vi "Cfg from FP.vi"(8 "error in (no error)":errorcluster, 11 "Measure Object in":refnum<class "Log Record.lvclass">) -> (0 "error out":errorcluster, 3 "Measure Object out":refnum<class "Log Record.lvclass">)   [LabVIEW 2020, in "Log Record.lvclass"]
uses:
  Template Module/Template Module.lvclass/Template Module.ctl
  Template Module/Write Configuration.vi
  Log Record.lvclass
  Process Object/Process Object.lvclass
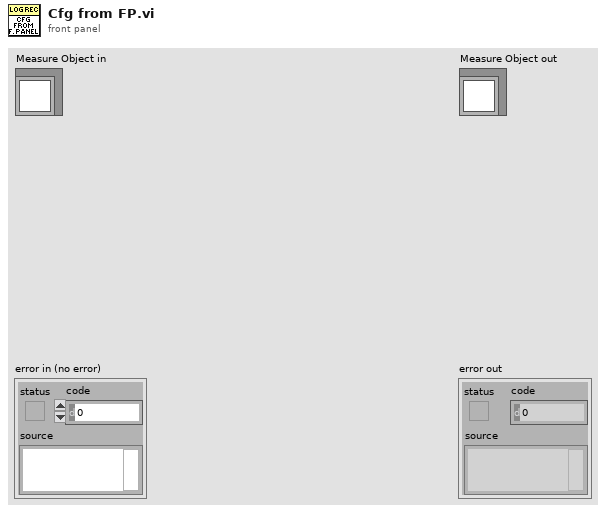
[diagram p1: front panel]
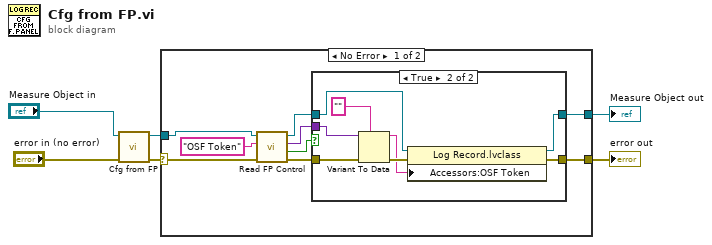
[diagram p0: block diagram]
diagram:
  n1 = call-parent "Cfg from FP.vi"("error in (no error)"="error in (no error)", "Measure Object in"="Measure Object in") -> ("error out"=w4:errorcluster, "Measure Object out"=w3:refnum<class "Log Record.lvclass">)  [unwired: 8 in]
  n2 = case shown="No Error" w4 {
    selector: w4 -> [w9 w27]
    tunnel: [w8 w27] -> w1
    tunnel: [w12 w26] -> w2
    tunnel: w3 -> [w15 w26]
    frame No Error {
      n3 = call-dynamic "Read FP Control.vi"("error in (no error)"=w9, "Control Name"="OSF Token", "Measure Object in"=w15) -> ("error out"=w10:errorcluster, "Present"=w7:bool, "Control Value"=w11:variant, "Measure Object out"=w14:refnum<class "Log Record.lvclass">)  [unwired: 5 in]
      n4 = case shown="True" w7 {
        tunnel: w14 -> [w16 w25]
        tunnel: [w16 w24] -> w12
        tunnel: w11 -> [_ w19]
        tunnel: w10 -> [w17 w23]
        tunnel: [w17 w22] -> w8
        frame False {
        }
        frame True {
          n5 = Variant To Data(error in=w23, type="", Variant=w19) -> (data=w20:string, error out=w21:errorcluster)
          n6 = property class="Log Record.lvclass"(reference=w25, error in=w21, "Accessors:OSF Token"=w20) -> (reference out=w24:refnum<class "Log Record.lvclass">, error out=w22:errorcluster)
        }
      }
    }
    frame Error {
    }
  }
  "error out" <- w1
  "Measure Object out" <- w2
